vi "Actor Core.vi"(8 "error in":errorcluster, 11 "Panel in":refnum<class "MiniGUI.lvclass">) -> (0 "error out":errorcluster, 3 "Actor out":refnum<class "Actor.lvclass">)   [LabVIEW 2019, in "MiniGUI.lvlib" / "MiniGUI.lvclass"]
doc: "Shows the Label and a log of all events for the panel.\n----\nCopyright: MGI 2016\nAuthor: Derek Trepanier"
uses:
  MiniGUI.lvclass
  C:/Program Files (x86)/National Instruments/LabVIEW 2019/vi.lib/MGI/Panel Manager/Panel Actor/Panel Actor/Panel Actor.lvclass
  <vilib>/ActorFramework/Actor/Actor.lvclass
  Dataset GUI.ctl
  MiniGUI.lvclass/MiniGUI.ctl
  LabGUI Head.ctl
  <vilib>/ActorFramework/Message Enqueuer/Message Enqueuer.lvclass/Message Enqueuer.ctl
  <vilib>/ActorFramework/Message Enqueuer/Enqueue.vi
  <vilib>/ActorFramework/Stop Msg/Stop Msg.lvclass
  C:/Program Files (x86)/National Instruments/LabVIEW 2019/vi.lib/ActorFramework/Message/Message.lvclass
  <vilib>/ActorFramework/Message Priority Queue/Priority Enqueue.vi
  <vilib>/MGI/Panel Manager/Panel Actor/Panel Actor/Panel Actor.lvclass
  MiniGUI.lvlib
panel:
  out "Title":string="SoftwareTest (192.168.1.109)"
  out "IP Address":string
  out "Compressor":bool=TRUE
  out "Dataset":T1={"M1 Status"={"Read Temp"=273.15, "Bin String"="", "M1 Set Temp"=273.15, "Feedback"=1}, "M2 Status"={"Read Temp"=273.15, "Bin String"="", "M2 Set Temp"=273.15, "Feedback"=1}} {"M2 Status"."Feedback" items=["Evap Temp", "Case Temp", "Intec Temp", "TSD  Temp", "Autotune", "Extra"]; "M2 Status"."M2 Set Temp" format="%.1f"; "M2 Status"."Read Temp" format="%.1f"; "M1 Status"."Feedback" items=["Evap Temp", "Case Temp", "Intec Temp", "TSD  Temp", "Autotune", "Extra"]; "M1 Status"."M1 Set Temp" format="%.1f"; "M1 Status"."Read Temp" format="%.1f"}
  out "Note":string="SoftwareTest (192.168.1.109)"
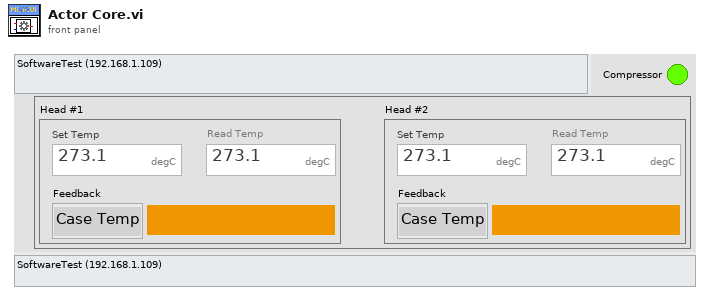
[diagram p1: front panel]
types:
  T1 = typedef "MiniGUI.lvlib/Dataset GUI.ctl" = cluster{"M1 Status":cluster{"Read Temp":dbl[unit], "Bin String":string, "M1 Set Temp":dbl[unit], "Feedback":u8}, "M2 Status":cluster{"Read Temp":dbl[unit], "Bin String":string, "M2 Set Temp":dbl[unit], "Feedback":u8}}
  T2 = enum32{"Invalid", "Standard", "Closed", "Hidden", "Minimized", "Maximized"}
  T3 = cluster{"MiniGUI Dataset":refnum<user-event>, "RT Dataset":refnum<user-event>}
  T4 = cluster{"Event Registration Refnum":refnum<event-registration>, "Pnl Actor":refnum<event-registration>}
  T5 = typedef "Panel.lvlib/Panel Helper.lvclass/Events.ctl" = enum16{"Initialized", "Shown", "Hidden", "Closed"}
  T6 = typedef "LabGUI Head.ctl" = cluster{"SV":dbl, "PV":dbl, "String":string, "Color Box":u32, "FeedBack":enum16{""}}
  T7 = cluster{"Read Temp":dbl[unit], "Bin String":string, "M1 Set Temp":dbl[unit], "Feedback":u8}
  T8 = cluster{"Read Temp":dbl[unit], "Bin String":string, "M2 Set Temp":dbl[unit], "Feedback":u8}
  T9 = typedef "MiniGUI.lvlib/MiniGUI.ctl" = cluster{"M1 Status":cluster{"Read Temp":dbl[unit], "Bin String":string, "M1 Set Temp":dbl[unit], "Feedback":u8}, "M2 Status":cluster{"Read Temp":dbl[unit], "Bin String":string, "M2 Set Temp":dbl[unit], "Feedback":u8}}
  T10 = cluster{"Compressor":bool, "M1":T6, "M2":T6, "Error":string, "System Name":string, "dual head":bool}
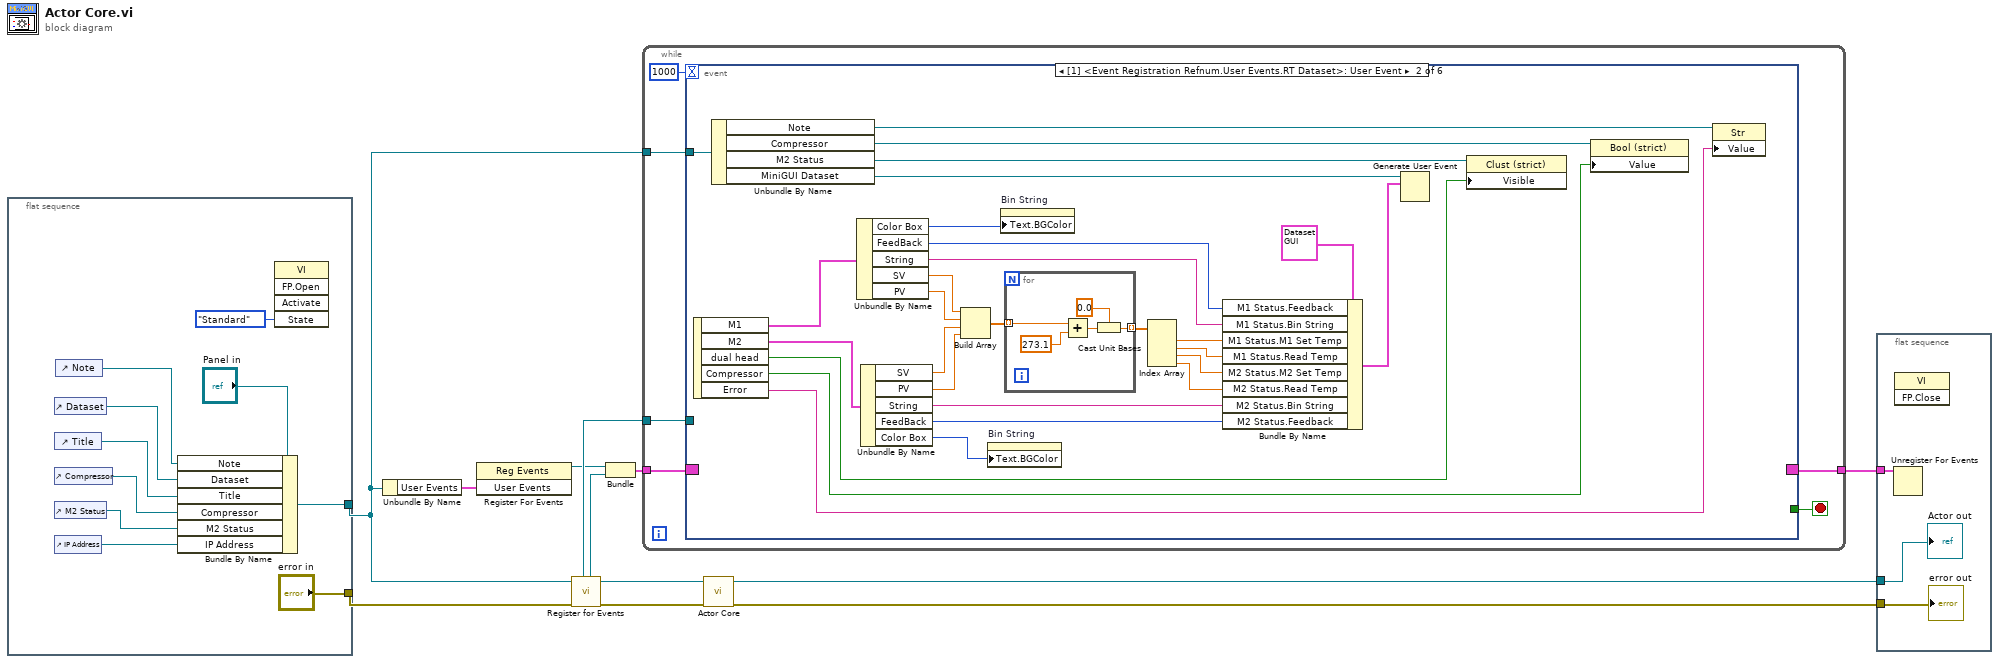
[diagram p0: block diagram]
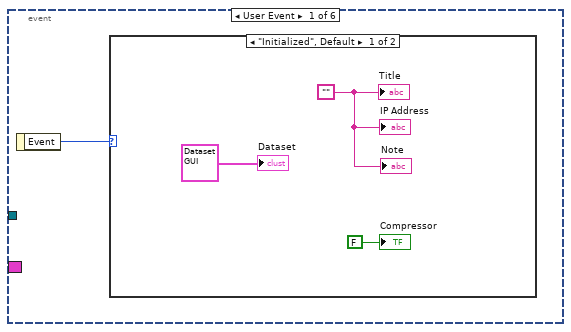
[diagram p2: hidden frame]
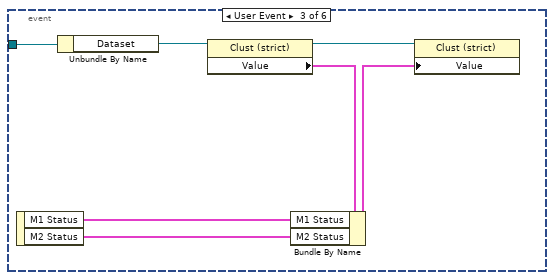
[diagram p4: hidden frame]
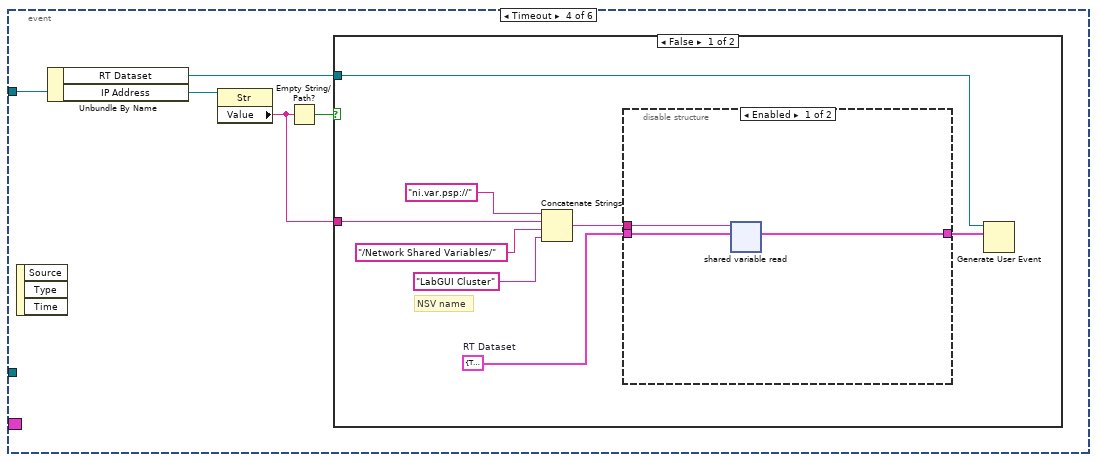
[diagram p5: hidden frame]
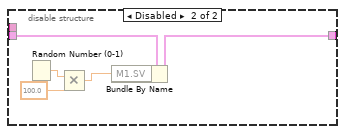
[diagram p6: hidden frame]
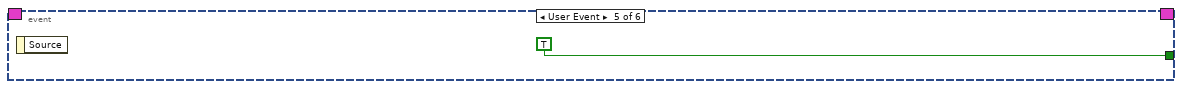
[diagram p8: hidden frame]
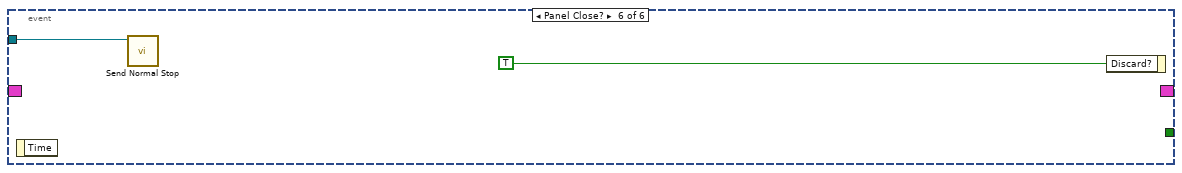
[diagram p9: hidden frame]
diagram:
  n1 = flat-sequence {
    tunnel: [w20] -> w1
    tunnel: ["error in"] -> w2
    frame #0 {
      n2 = control-ref of="Dataset"() -> (w15:refnum<vi>)
      n3 = control-ref of="Title"() -> (w16:refnum<vi>)
      n4 = control-ref of="Compressor"() -> (w18:refnum<vi>)
      n5 = control-ref of="M2 Status"() -> (w14:refnum<vi>)
      n6 = control-ref of="IP Address"() -> (w17:refnum<vi>)
      n7 = control-ref of="Note"() -> (w13:refnum<vi>)
      n8 = Bundle By Name(cluster="Panel in", "Note"=w13, "Dataset"=w15, "Title"=w16, "Compressor"=w18, "M2 Status"=w14, "IP Address"=w17) -> (w20:refnum<class "MiniGUI.lvclass">)
      n9 = invoke class="VI" method="FP.Open"("State"=T2."Standard") -> ()  [unwired: 4 in, 5 out]
    }
  }
  n10 = Unbundle By Name(w1) -> ("User Events"=w4:T3)
  n11 = register-events(w4) -> (reference out=w3:refnum<event-registration>)  [unwired: 2 in, 1 out]
  n12 = call <vilib>:"Register for Events.vi"("Error In"=w2, "Panel Actor in"=w1) -> ("Error Out"=w10:errorcluster, "Panel Actor out"=w12:refnum<class "MiniGUI.lvclass">, "Pnl Actor"=w6:refnum<event-registration>, "Self Enqueuer"=w11:refnum<class "Message Enqueuer.lvclass">)  [unwired: 6 in]
  n13 = Bundle("Event Registration Refnum"=w3, "Pnl Actor"=w6) -> (w5:T4)  [unwired: 1 in]
  n14 = while {
    tunnel: w11 -> [w28]
    tunnel: w5 -> [w24]
    tunnel: [w26] -> w9
    tunnel: w1 -> [w25]
    stop <- w27 stop-if-true
    n15 = event shown="[1] <Event Registration Refnum.User Events.RT Dataset>: User Event" {
      selector: w24 -> [_ _ _ _ _ _]
      dyn-events: [_ _ _ _ _ _] -> w26
      timeout: 1000 -> [_ _ _ _ _ _]
      tunnel: w28 -> [_ _ _ _ _ w95]
      tunnel: [_ _ _ _ TRUE _] -> w27
      tunnel: w25 -> [_ w60 w72 w77 _ _]
      event User Event {
        n16 = event-data() -> ("Event"=w29:T5)  [unwired: 1 in]
        n17 = case shown="\"Initialized\", Default" w29 {
          frame "Initialized", Default {
            w31 = ""
            "IP Address" <- w31
            "Title" <- w31
            "Compressor" <- FALSE ("Connect")
            "Note" <- w31
            "Dataset" <- T1 {"M1 Status"={"Read Temp"=273.15, "Bin String"="", "M1 Set Temp"=273.15, "Feedback"=1}, "M2 Status"={"Read Temp"=273.15, "Bin String"="", "M2 Set Temp"=273.15, "Feedback"=1}} ("Dataset")
          }
          frame "Shown" {
          }
        }
      }
      event User Event {
        n18 = event-data() -> ("M1"=w49:T6, "M2"=w43:T6, "dual head"=w50:bool, "Compressor"=w51:bool, "Error"=w52:string)  [unwired: 1 in]
        n19 = Unbundle By Name(w60) -> ("Note"=w53:refnum<vi>, "Compressor"=w54:refnum<vi>, "M2 Status"=w55:refnum<vi>, "MiniGUI Dataset"=w59:refnum<user-event>)
        n20 = Unbundle By Name(w49) -> ("Color Box"=w33:u32, "FeedBack"=w34:enum16{""}, "String"=w35:string, "SV"=w48:dbl, "PV"=w47:dbl)
        n21 = Unbundle By Name(w43) -> ("SV"=w46:dbl, "PV"=w45:dbl, "String"=w38:string, "FeedBack"=w37:enum16{""}, "Color Box"=w36:u32)
        n22 = Build Array(w48, w47, w46, w45) -> (w44:dbl[])
        n23 = property on="Bin String" class="Str"("Text.BGColor"=w36) -> ()  [unwired: 2 in, 2 out]
        n24 = property on="Bin String" class="Str"("Text.BGColor"=w33) -> ()  [unwired: 2 in, 2 out]
        n25 = for {
          tunnel: w44 -> [w62] mode=indexing
          tunnel: [w64] -> w58 mode=indexing
          n26 = Add(x=w62, y=273.1) -> (x+y=w63:dbl)
          n27 = Cast Unit Bases(0:w63, 1:dbl[unit] 0.0 ("M1 Status.Read Temp")) -> (2:w64:dbl[unit])
        }
        n28 = Index Array(array=w58) -> (element #1=w42:dbl[unit], element #2=w41:dbl[unit], element #3=w40:dbl[unit], element #4=w39:dbl[unit])  [unwired: 4 in]
        n29 = Bundle By Name(cluster=T1 {"M1 Status"={"Read Temp"=393.25, "Bin String"="", "M1 Set Temp"=393.65, "Feedback"=1}, "M2 Status"={"Read Temp"=393.25, "Bin String"="", "M2 Set Temp"=393.65, "Feedback"=1}} ("Value"), "M1 Status.Feedback"=w34, "M1 Status.Bin String"=w35, "M1 Status.M1 Set Temp"=w42, "M1 Status.Read Temp"=w41, "M2 Status.M2 Set Temp"=w40, "M2 Status.Read Temp"=w39, "M2 Status.Bin String"=w38, "M2 Status.Feedback"=w37) -> (w56:T1)
        n30 = Generate User Event(user event=w59, event data cluster=w56) -> ()  [unwired: 2 in, 2 out]
        n31 = property class="Clust (strict)"(reference=w55, "Visible"=w50) -> ()  [unwired: 1 in, 2 out]
        n32 = property class="Bool (strict)"(reference=w54, "Value"=w51) -> ()  [unwired: 1 in, 2 out]
        n33 = property class="Str"(reference=w53, "Value"=w52) -> ()  [unwired: 1 in, 2 out]
      }
      event User Event {
        n34 = event-data() -> ("M1 Status"=w67:T7, "M2 Status"=w66:T8)  [unwired: 1 in]
        n35 = Unbundle By Name(w72) -> ("Dataset"=w70:refnum<vi>)
        n36 = property class="Clust (strict)"(reference=w70) -> (reference out=w71:refnum<vi>, "Value"=w69:T9)  [unwired: 1 in, 1 out]
        n37 = Bundle By Name(cluster=w69, "M1 Status"=w67, "M2 Status"=w66) -> (w68:T9)
        n38 = property class="Clust (strict)"(reference=w71, "Value"=w68) -> ()  [unwired: 1 in, 2 out]
      }
      event Timeout {
        n39 = event-data() -> ()  [unwired: 1 in, 3 out]
        n40 = Unbundle By Name(w77) -> ("RT Dataset"=w74:refnum<user-event>, "IP Address"=w76:refnum<vi>)
        n41 = property class="Str"(reference=w76) -> ("Value"=w73:string)  [unwired: 1 in, 2 out]
        n42 = Empty String/Path?(string/path=w73) -> (empty?=w75:bool)
        n43 = case shown="False" w75 {
          tunnel: w74 -> [w82 _]
          tunnel: w73 -> [w78 _]
          frame False {
            w79 = T10 {"Compressor"=TRUE, "M1"={"SV"=100.0, "PV"=200.0, "String"="", "Color Box"=6618880, "FeedBack"=enum.""}, "M2"={"SV"=300.0, "PV"=400.0, "String"="", "Color Box"=16725248, "FeedBack"=enum.""}, "Error"="", "System Name"="", "dual head"=TRUE}  # RT Dataset
            # "NSV name"
            n44 = Concatenate Strings("ni.var.psp://", w78, "/Network Shared Variables/", "LabGUI Cluster") -> (w80:string)
            n45 = disable-structure shown="Enabled" {
              disable-tunnel: [w88 w92] -> w81
              disable-tunnel: w80 -> [w87 _]
              disable-tunnel: w79 -> [w86 w93]
              frame Enabled {
                n46 = shared-variable-read(w87, w86) -> (w88:T10)  [unwired: 1 in, 3 out]
              }
              frame Disabled {
                n47 = Random Number (0-1)() -> (number: 0 to 1=w91:dbl)
                n48 = Multiply(x=w91, y=100.0) -> (x*y=w89:dbl)
                n49 = Bundle By Name(cluster=w93, "M1.SV"=w89) -> (w92:T10)
              }
            }
            n50 = Generate User Event(user event=w82, event data cluster=w81) -> ()  [unwired: 2 in, 2 out]
          }
          frame True {
          }
        }
      }
      event User Event {
        n51 = event-data() -> ()  [unwired: 1 in, 1 out]
      }
      event Panel Close? {
        n52 = event-data() -> ()  [unwired: 1 in, 1 out]
        n53 = call <vilib>:"Send Normal Stop.vi"("Message Enqueuer"=w95) -> ()  [unwired: 10 in, 1 out]
        n54 = event-data("Discard?"=TRUE) -> ()  [unwired: 1 in, 1 out]
      }
    }
  }
  n55 = call-parent "Actor Core.vi"("error in"=w10, "Panel Actor in"=w12) -> ("error out"=w7:errorcluster, "Actor out"=w8:refnum<class "Actor.lvclass">)  [unwired: 8 in]
  n56 = flat-sequence {
    tunnel: w9 -> [w99]
    tunnel: w8 -> [w98]
    tunnel: w7 -> [w97]
    frame #0 {
      n57 = Unregister For Events(event registration refnum=w99) -> ()  [unwired: 1 in, 1 out]
      n58 = invoke class="VI" method="FP.Close"() -> ()  [unwired: 3 in, 3 out]
      "error out" <- w97
      "Actor out" <- w98
    }
  }
